vi "Wind_Tunnel_Main.vi"() -> ()   [LabVIEW 2025]
uses:
  <vilib>/express/express arith-compare/Formula/XNode/ExpressFormulaBlockNode.xnode
  <vilib>/ptbypt/NI_PtbyPt.lvlib
panel:
  out "LC2":dbl
  out "LC0":dbl
  out "LC1":dbl
  out "Voltage Out":dbl
  out "FRQ":dbl
  out "P10(AS1)":dbl
  out "P9":dbl
  out "P8":dbl
  out "P7":dbl
  out "P6":dbl
  out "P5(AS0)":dbl
  out "P4":dbl
  out "P3":dbl
  out "P2":dbl
  out "P1":dbl
  out "Drag (N)":dbl
  in  "Sting Angle":dbl
  out "LC2 (N)":dbl format="%#_4g"
  out "LC1 (N)":dbl format="%#_4g"
  out "LC0 (N)":dbl format="%#_4g"
  in  "Spreadsheet Path":path=path "C:/Users/student/Desktop/Wind Tunnel Software/Testing Data"
  out "Lift (N)":dbl
  out "Estimated Velocity (m/s)":dbl
  in  "Single Shot":bool
  in  "Spreadsheet Name. (Needs to end in \".csv\")":string="%Y-%m-%d_%H-%M-%S.csv"
  out "ESTOP ACTIVE":bool
  in  "ESTOP":bool
  in  "SYSTEM TARE":bool
  in  "Tare LC0":bool
  out "?":dbl
  out "LC0 (N)":dbl(graph)
  in  "Tare LC1":bool
  out "?":dbl
  out "LC1 (N)":dbl(graph)
  in  "Tare LC2":bool
  in  "Tare Pitot Tube\nNote: ONLY USE AT\nIDLE":bool
  out "?":dbl
  out "LC2 (N)":dbl(graph)
  out "?":bool
  out "?":bool
  in  "VFD \nMode\nSelect":bool=TRUE
  out "VFD Frequency (Hz)":dbl
  in  "Speed %\n0-100":dbl min=0.0 max=100.0
  in  "Target Speed (m/s)":dbl min=0.0 max=100.0
  out "V_DIFF":dbl
  out "Dynamic Voltage":dbl format="%0.2f"
  out "Static Voltage":dbl format="%0.2f"
  in  "Enable Data Collection\n(Excel Spreadsheet)":bool caption="Enable"
  out "?":bool
  out "Airspeed Warning Indicator":string
  out "IAS (m/s)":dbl format="%#_4g"
  out "Indicated Velocity Graph (m/s)":dbl(graph)
  in  "System Stop":bool=TRUE
  # "System Controls"
  # "Wind Tunnel Data"
  # "Quick Start"
  # "Raw Voltage Data"
  # "0. Read the Documentation!!!\n1. Familiarize yourself with this panel. Pressing Ctrl+H will bring up a help menu. Hovering over components will bring up more information.\n2.Looking at the graphs, they will not be zeroed\nTo fix this press SYSTEM TARE (bottom right of this Panel).  You should expect the graphs to the right to be within +- 5 of zero after tare. \n3. Looking at the VFD box (the one attached to \nthe fan with dials/switches) make sure it is set\nto ON, switched to Automated, and check that the Emergency Stop button is not pressed. If it is, twist it clockwise to reset"
  # "4. Now the fan is controlled by this panel. On the\n\"Fan Controls\" below, set the \"VFD mode switch\" to the upward postition to to enable Speed % Mode, which controls the fan by a percentage of its maximum power. You can now adjust the box \"Speed %\" which will spin up the fan.\n\nNOTE:  To save data to CSV, first hit \"System Stop\", then refer to the controls on the bottom of this panel. Select the Enable Data Collection button so it displays \"Enabled\". Then set the Spreadsheet Path by selecting the little folder icon and following the prompts. Change the name as desired. Start over from step 0"
  # "Pitot Tube\nControls"
  # "Shutdown Procedure"
  # "Fan Controls"
  # "1. Set both speed % and target speed controls to 0. Wait for fan to spin down\n2. Press system stop.\n3. On the VFD, set the switch to \"MANUAL\", press the physical E-Stop, make sure dial is set to 0, and then set the switch to \"OFF \".\n4. Set the switch on the power box to the downward off position and lock.\n5. Unplug the black powerstrip behind this computer"
  # "Measurements inaccurate under 10m/s"
  # "MAX 100"
  # "MAX 70"
  # "System Controls"
  # "IGNORE THESE, not accurate\n <--- No correction factor"
  # "Derived Values:"
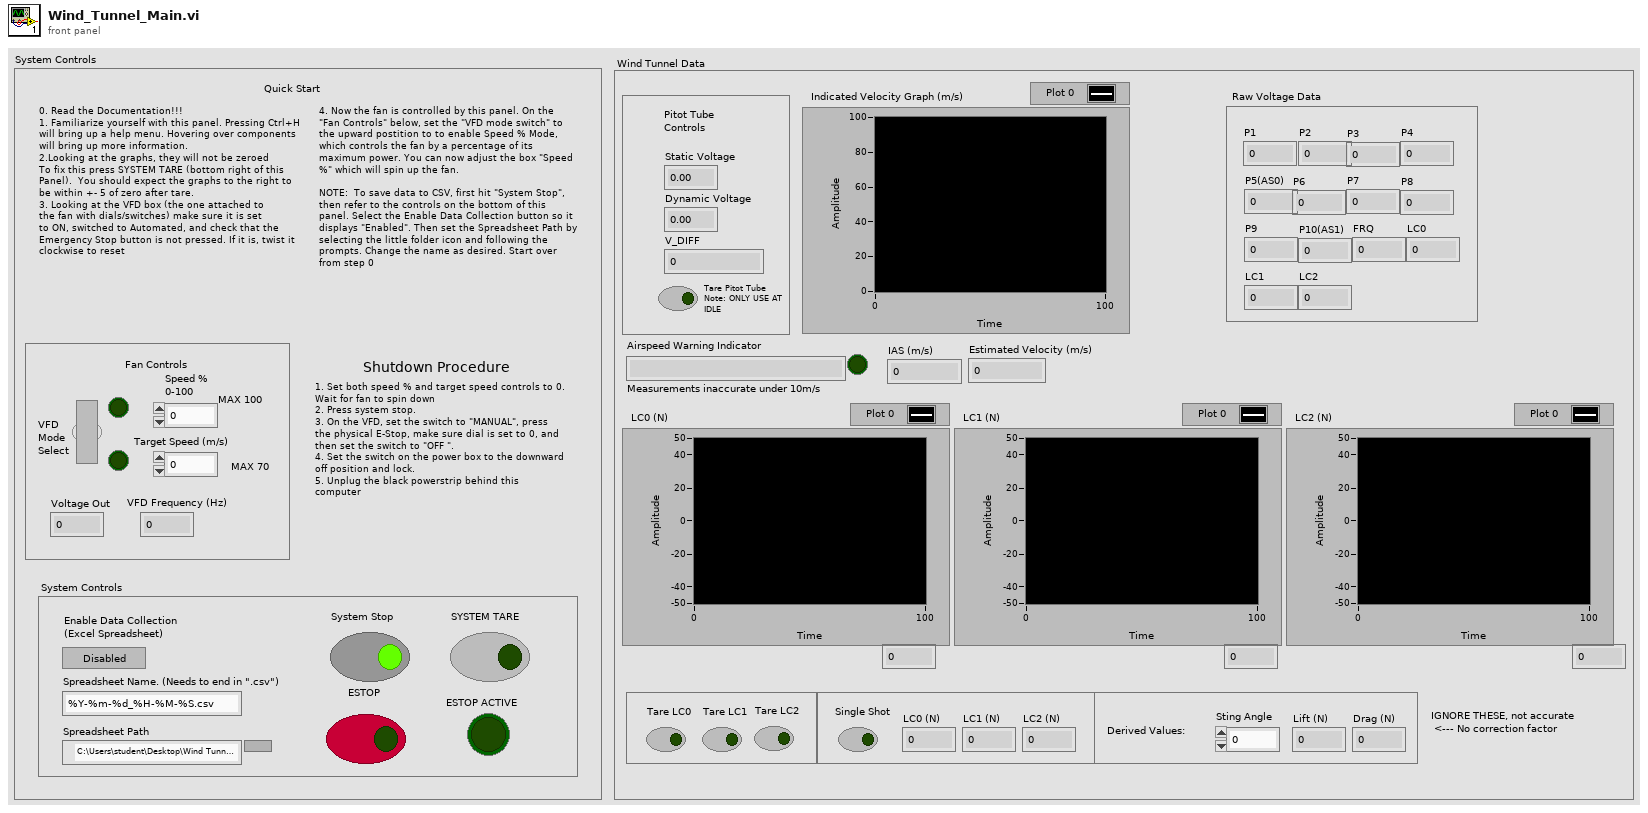
[diagram p1: front panel]
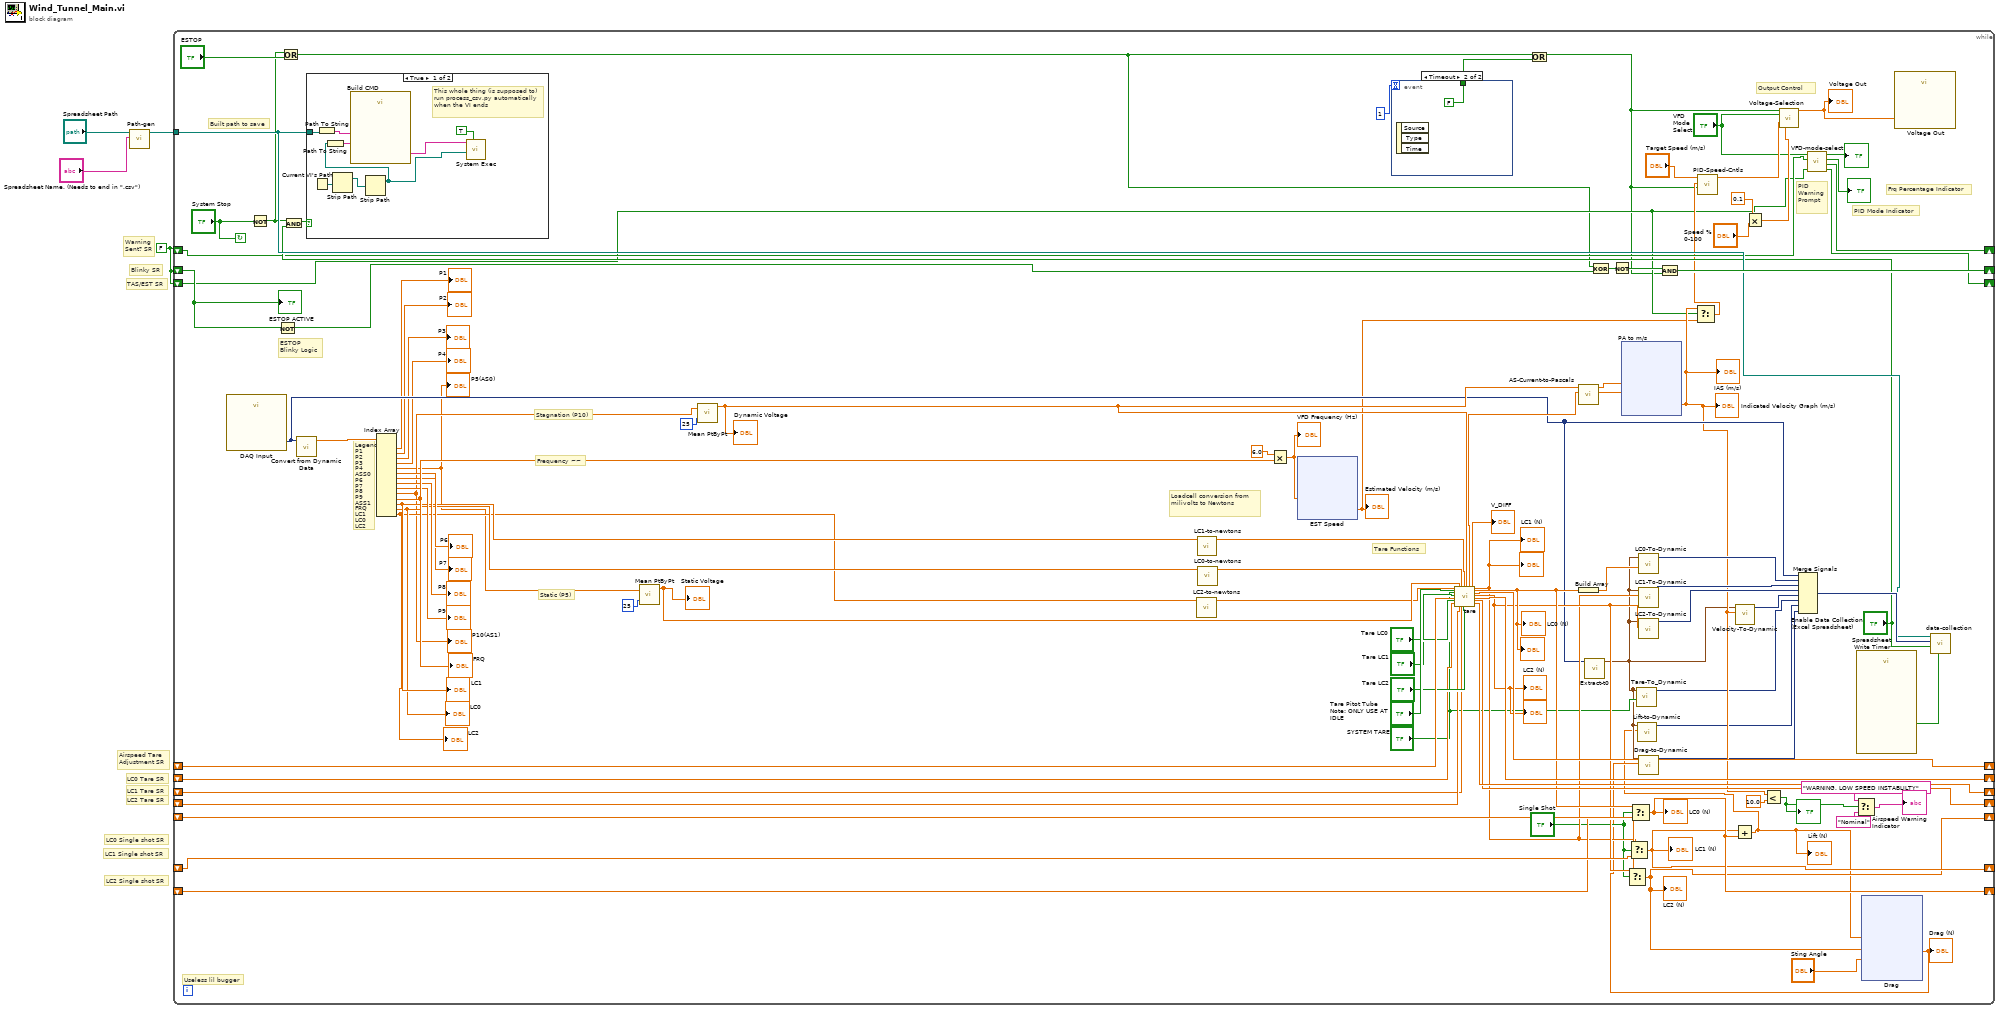
[diagram p0: block diagram]
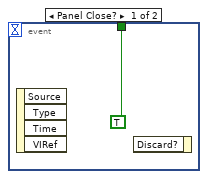
[diagram p2: hidden frame]
diagram:
  w1 = FALSE
  # "TAS/EST SR"
  # "LC2 Tare SR"
  # "LC2 Single shot SR"
  # "LC1 Single shot SR"
  # "LC0 Single shot SR"
  # "LC1 Tare SR"
  # "LC0 Tare SR"
  # "Airspeed Tare\nAdjustment SR"
  # "Warning\nSent? SR"
  # "Blinky SR"
  n1 = call "Path-gen.vi"("Spreadsheet Name"="Spreadsheet Name. (Needs to end in \".csv\")", "Spreadsheet Path"="Spreadsheet Path") -> ("appended path"=w4:path)  [unwired: 9 in]
  n2 = while {
    tunnel: w4 -> [w39]
    shift-right: [w93] -> _
    shift-left: _ -> [w94]
    shift-right: [w80] -> _
    shift-left: _ -> [w89]
    shift-right: [w84] -> _
    shift-left: _ -> [w90]
    shift-right: [w82] -> _
    shift-left: _ -> [w46]
    shift-right: [w75] -> _
    shift-left: w1 -> [w77]
    shift-right: [w27] -> _
    shift-left: w1 -> [w30]
    shift-right: [w59] -> _
    shift-left: _ -> [w71]
    shift-right: [w58] -> _
    shift-left: _ -> [w73]
    shift-right: [w57] -> _
    shift-left: _ -> [w72]
    shift-right: [w26] -> _
    shift-left: w1 -> [w23]
    stop <- "System Stop" continue-if-true
    # "Loadcell conversion from\nmilivolts to Newtons"
    # "Tare Functions"
    # "Built path to save"
    # "Useless lil bugger"
    # "Frequency ~~"
    # "Static (P5)"
    # "Stagnation (P10)"
    # "ESTOP\nBlinky Logic"
    # "Frq Percentage Indicator"
    # "PID Mode Indicator"
    # "PID \nWarning\nPrompt"
    # "Output Control"
    # "Legend\nP1\nP2\nP3\nP4\nASS0\nP6\nP7\nP8\nP9\nASS1\nFRQ\nLC1\nLC0\nLC2"
    n3 = call "DAQ Input"() -> ("data"=w61:dynamicdata)  [unwired: 16 in, 3 out]
    n4 = Not(x="System Stop") -> (.not. x?=w19:bool)
    n5 = Not(x=w77) -> (.not. x?=w76:bool)
    n6 = Or(x=w19, y="ESTOP") -> (x .or. y?=w20:bool)
    n7 = And(x=w19, y="Enable Data Collection\n(Excel Spreadsheet)") -> (x .and. y?=w33:bool)
    n8 = call "Convert from Dynamic Data"("Dynamic Data Type"=w61) -> ("Array"=w106:dbl[])  [unwired: 3 in]
    n9 = case shown="True" w33 {
      tunnel: w39 -> [w128 _]
      frame True {
        # "This whole thing (is supposed to) run process_csv.py automatically when the VI ends"
        n10 = Current VI's Path() -> (path=w125:path)
        n11 = Path To String(path=w128) -> (string=w124:string)
        n12 = Strip Path(path=w125) -> (stripped path=w122:path)  [unwired: 1 out]
        n13 = Strip Path(path=w122) -> (stripped path=w121:path)  [unwired: 1 out]
        n14 = Path To String(path=w121) -> (string=w123:string)
        n15 = call "Build CMD"("curdir"=w123, "s"=w124) -> ("Result"=w127:string)  [unwired: 12 in, 1 out]
        n16 = call <vilib>:"System Exec.vi"("wait until completion? (T)"=TRUE, "working directory"=w121, "command line"=w127) -> ()  [unwired: 5 in, 4 out]
      }
      frame False {
      }
    }
    n17 = Index Array(array=w106) -> (element #1=→"P1":dbl, element #2=→"P2":dbl, element #3=→"P3":dbl, element #4=→"P4":dbl, element #5=w41:dbl, element #6=→"P6":dbl, element #7=→"P7":dbl, element #8=→"P8":dbl, element #9=→"P9":dbl, element #10=w42:dbl, element #11=w95:dbl, element #12=w45:dbl, element #13=w44:dbl, element #14=w43:dbl)  [unwired: 14 in]
    "P5(AS0)" <- w41
    "P10(AS1)" <- w42
    "FRQ" <- w95
    "LC1" <- w45
    "LC0" <- w44
    "LC2" <- w43
    n18 = call <vilib>:"Mean PtByPt.vi"("x"=w41, "sample length"=25) -> ("mean"=w103:dbl)  [unwired: 2 in, 1 out]
    "Static Voltage" <- w103
    n19 = call <vilib>:"Mean PtByPt.vi"("x"=w42, "sample length"=25) -> ("mean"=w102:dbl)  [unwired: 2 in, 1 out]
    "Dynamic Voltage" <- w102
    n20 = call "LC2-to-newtons.vi"("mv in"=w43) -> ("newtons out"=w79:dbl)  [unwired: 10 in]
    n21 = call "LC1-to-newtons.vi"("LC In"=w45) -> ("Newtons Out"=w83:dbl)  [unwired: 10 in]
    n22 = call "LC0-to-newtons.vi"("mv in"=w44) -> ("newtons out"=w81:dbl)  [unwired: 10 in]
    n23 = Multiply(x=6.0, y=w95) -> (x*y=w60:dbl)
    "VFD Frequency (Hz)" <- w60
    n24 = xnode "EST Speed"("X1"=w60) -> ("Result"=w22:dbl)  [unwired: 1 in, 1 out]
    "Estimated Velocity (m/s)" <- w22
    n25 = event shown="[1] Timeout" {
      selector: _ -> [_ _]
      dyn-events: _ -> [_ _]
      timeout: 1 -> [_ _]
      tunnel: [TRUE FALSE] -> w11
      event Panel Close? {
        n26 = event-data() -> ()  [unwired: 1 in, 4 out]
        n27 = event-data() -> ()  [unwired: 2 in, 1 out]
      }
      event Timeout {
        n28 = event-data() -> ()  [unwired: 1 in, 3 out]
      }
    }
    n29 = call "tare.vi"("LC2 Tare\nAmount"=w79, "Tare Pitot Tube\nNote: ONLY USE AT\nIDLE"="Tare Pitot Tube\nNote: ONLY USE AT\nIDLE", "SYSTEM TARE\nONLY USE AT IDLE"="SYSTEM TARE", "Tare LC1"="Tare LC1", "Previous \nAdjustment"=w94, "Tare LC0"="Tare LC0", "LC0 Prev"=w90, "AS 0"=w103, "LC2 Prev"=w89, "LC1 Tare \nAmount"=w81, "LC1 Prev"=w46, "LC0 Tare\nAmount"=w83, "Tare LC2"="Tare LC2", "AS 1"=w102) -> ("AS0 Out"=w101:dbl, "V_DIFF\nIndicator"=→"V_DIFF":dbl, "LC1 Out"=w67:dbl, "LC0 Out"=w69:dbl, "Adjustment To Shift"=w93:dbl, "LC2 Out"=w68:dbl, "LC0 To\nShift"=w84:dbl, "LC2 To \nShift"=w80:dbl, "LC1 to \nShift"=w82:dbl)  [unwired: 5 in]
    "LC2 (N)" <- w68
    "?" <- w68
    "LC1 (N)" <- w67
    "?" <- w67
    "LC0 (N)" <- w69
    "?" <- w69
    n30 = Or(x=w20, y=w11) -> (x .or. y?=w12:bool)
    n31 = call "AS-Current-to-Pascals.vi"("V0 In"=w101, "V1 In"=w102) -> ("PA1 Out"=w105:dbl, "PA0 Out"=w99:dbl)  [unwired: 8 in]
    n32 = Build Array(w69) -> (w65:dbl[])
    n33 = call "Extract-t0.vi"("data"=w61) -> ("Waveform"=w9:waveform(dbl))  [unwired: 10 in]
    n34 = Exclusive Or(1:w76, 2:w20) -> (0:w78:bool)
    n35 = Not(x=w78) -> (.not. x?=w74:bool)
    n36 = xnode ("PA to m/s")("pa0"=w99, "pa1"=w105) -> ("Result"=w25:dbl)  [unwired: 1 in, 1 out]
    "Indicated Velocity Graph (m/s)" <- w25
    "IAS (m/s)" <- w25
    n37 = Select(t=w68, s="Single Shot", f=w72) -> (s? t:f=w57:dbl)
    "LC2 (N)" <- w57
    n38 = Select(t=w67, s="Single Shot", f=w73) -> (s? t:f=w58:dbl)
    "LC1 (N)" <- w58
    n39 = Select(t=w69, s="Single Shot", f=w71) -> (s? t:f=w59:dbl)
    "LC0 (N)" <- w59
    n40 = call "Tare-To_Dynamic.vi"("Tare In"="SYSTEM TARE", "Waveform"=w9) -> ("Dynamic Data Type"=w17:dynamicdata)  [unwired: 9 in]
    n41 = call "LC0-To-Dynamic.vi"("Array"=w65, "Waveform"=w9) -> ("Dynamic Data Type"=w64:dynamicdata)  [unwired: 9 in]
    n42 = call "LC1-To-Dynamic.vi"("Numeric"=w67, "Waveform"=w9) -> ("Dynamic Data Type"=w62:dynamicdata)  [unwired: 9 in]
    n43 = call "LC2-To-Dynamic.vi"("Numeric"=w68, "Waveform"=w9) -> ("Dynamic Data Type"=w63:dynamicdata)  [unwired: 9 in]
    n44 = And(x=w74, y=w12) -> (x .and. y?=w75:bool)
    n45 = Select(t=w25, s=w23, f=w22) -> (s? t:f=w24:dbl)
    n46 = call "PID-Speed-Cntls.vi"("ESTOP"=w12, "PID IN"=w24, "Target Speed (m/s)"="Target Speed (m/s)") -> ("output"=w37:dbl)  [unwired: 8 in]
    n47 = call "Velocity-To-Dynamic.vi"("Result"=w25, "Waveform"=w9) -> ("Dynamic Data Type"=w66:dynamicdata)  [unwired: 9 in]
    n48 = Add(x=w58, y=w59) -> (x+y=w7:dbl)
    "Lift (N)" <- w7
    n49 = call "Lift-to-Dynamic.vi"("Lift In"=w7, "Waveform"=w9) -> ("Dynamic Data Type"=w6:dynamicdata)  [unwired: 9 in]
    n50 = Multiply(x=0.1, y="Speed %\n0-100") -> (x*y=w36:dbl)
    n51 = Less?(x=w25, y=10.0) -> (x < y?=w14:bool)
    "?" <- w14
    n52 = call "Voltage-Selection.vi"("ESTOP"=w12, "VFD \nMode\nSelect"="VFD \nMode\nSelect", "PID In"=w37, "Percentage\nIn"=w36) -> ("output"=w34:dbl)  [unwired: 11 in]
    "Voltage Out" <- w34
    n53 = call "VFD-mode-select.vi"("Est/TAS IN"=w23, "Warning\nSent? IN"=w30, "VFD \nMode\nSelect"="VFD \nMode\nSelect") -> ("EST/TAS out"=w26:bool, "Warning\nSent? OUT"=w27:bool, "PID Mode Indc"=→"?":bool, "FRQ Indc"=→"?":bool)  [unwired: 5 in]
    n54 = call "Spreadsheet Write Timer"() -> ("Time has Elapsed"=w100:bool)  [unwired: 12 in, 7 out]
    n55 = Select(t="WARNING. LOW SPEED INSTABLILTY", s=w14, f="Nominal") -> (s? t:f=→"Airspeed Warning Indicator":string)
    n56 = xnode "Drag"("L"=w7, "LC2"=w57, "theta"="Sting Angle") -> ("Result"=w8:dbl)  [unwired: 1 in, 1 out]
    "Drag (N)" <- w8
    n57 = call "Drag-to-Dynamic.vi"("Drag In"=w8, "Waveform"=w9) -> ("Dynamic Data Type"=w5:dynamicdata)  [unwired: 9 in]
    n58 = Merge Signals(w61, w64, w62, w63, w66, w17, w6, w5) -> (w70:dynamicdata)
    n59 = call "Voltage Out"("data"=w34) -> ()  [unwired: 17 in, 2 out]
    n60 = call "data-collection.vi"("Time has Elapsed"=w100, "Enable Data Collection\n(Excel Spreadsheet)"="Enable Data Collection\n(Excel Spreadsheet)", "Dynamic Data"=w70, "appended path"=w39) -> ()  [unwired: 8 in]
    "ESTOP ACTIVE" <- w77
  }
